vi "CallVirtualConstructorMethod.vi"(8 "error in":errorcluster, 11 "TestSuite in":refnum<class "TestSuite.lvclass">) -> (0 "error out":errorcluster, 2 "Constructor Error":errorcluster, 3 "TestSuite out":refnum<class "TestSuite.lvclass">)   [LabVIEW 2011, in "TestSuite.lvclass"]
uses:
  TestSuite.lvclass
  JKI Reuse/Filter Error Codes (Scalar)__jki_lib_error_handling -- VI Tester.vi
  Libraries/VITesterUtilities.lvlib
panel:
  # "JKI VI Tester for LabVIEW\nhttp://jkisoft.com/vi-tester\nCopyright (C) 2007-2009, JKI <info@jkisoft.com>\nALL RIGHTS RESERVED"
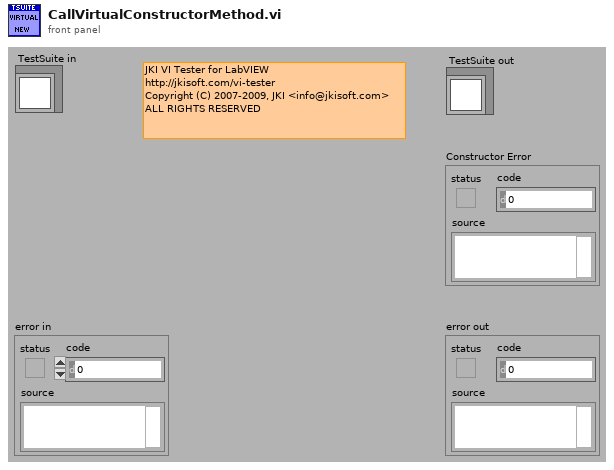
[diagram p1: front panel]
types:
  T1 = cluster{"name":string, "type desc":i16[], "flat data":string}
  T2 = cluster{"name":string, "type desc":i16[], "flat data":string}[]
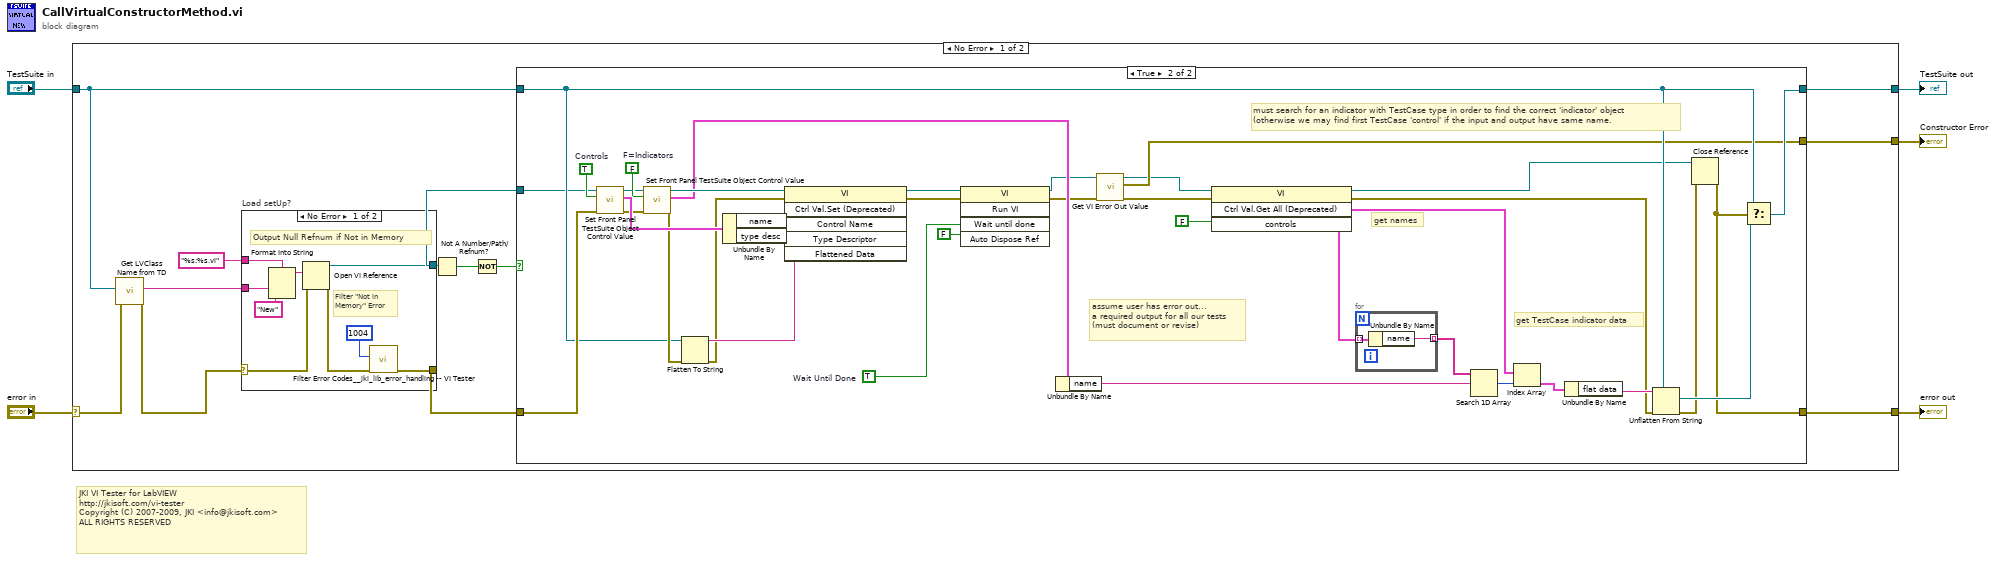
[diagram p0: block diagram]
diagram:
  # "JKI VI Tester for LabVIEW\nhttp://jkisoft.com/vi-tester\nCopyright (C) 2007-2009, JKI <info@jkisoft.com>\nALL RIGHTS RESERVED"
  n1 = case shown="No Error" "error in" {
    selector: "error in" -> [w11 w70]
    tunnel: [w17 w69] -> w1
    tunnel: [w16 _] -> w2
    tunnel: [w15 w70] -> w3
    tunnel: "TestSuite in" -> [w12 w69]
    frame No Error {
      n2 = call "Get LVClass Name from TD.vi"("error in"=w11, "Variant"=w12) -> ("error out"=w10:errorcluster, "LVClass Name"=w13:string)  [unwired: 8 in]
      n3 = case "Load setUp?" shown="No Error" w10 {
        selector: w10 -> [w21 w27]
        tunnel: [w24 _] -> w6
        tunnel: "%s:%s.vi" ("format string") -> [w23 _]
        tunnel: [w19 w27] -> w9
        tunnel: w13 -> [w22 _]
        frame No Error {
          # "Output Null Refnum if Not in Memory"
          # "Filter \"Not in Memory\" Error"
          n4 = Format Into String(format string=w23, w22, "New" ("input 2")) -> (resulting string=w25:string)  [unwired: 2 in, 1 out]
          n5 = Open VI Reference(vi path=w25, error in (no error)=w21) -> (vi reference=w24:refnum<vi>, error out=w20:errorcluster)  [unwired: 4 in]
          n6 = call-poly "Filter Error Codes__jki_lib_error_handling -- VI Tester.vi"("error in"=w20, "error code to filter"=1004) -> ("error out"=w19:errorcluster)  [unwired: 7 in, 2 out]
        }
        frame Error {
        }
      }
      n7 = Not A Number/Path/Refnum?(number/path/refnum=w6) -> (NaN/Path/Refnum?=w8:bool)
      n8 = Not(x=w8) -> (.not. x?=w7:bool)
      n9 = case shown="True" w7 {
        tunnel: [w29 w66] -> w17
        tunnel: [_ w32] -> w16
        tunnel: [w28 w36] -> w15
        tunnel: w12 -> [w29 w46]
        tunnel: w9 -> [w28 w54]
        tunnel: w6 -> [_ w35]
        frame False {
        }
        frame True {
          w51 = TRUE  # Wait Until Done
          w58 = FALSE  # F=Indicators
          w62 = TRUE  # Controls
          # "get TestCase indicator data"
          # "get names"
          # "must search for an indicator with TestCase type in order to find the correct 'indicator' object\n(otherwise we may find first TestCase 'control' if the input and output have same name."
          # "assume user has error out...\na required output for all our tests\n(must document or revise)"
          n10 = call "Set Front Panel TestSuite Object Control Value.vi"("error in"=w54, "Control (F: Indicator)"=w62, "vi reference"=w35) -> ("error out"=w57:errorcluster, "Control Value"=w61:T1, "dup vi reference"=w56:refnum<vi>)  [unwired: 5 in, 1 out]
          n11 = call "Set Front Panel TestSuite Object Control Value.vi"("error in"=w57, "Control (F: Indicator)"=w58, "vi reference"=w56) -> ("error out"=w53:errorcluster, "Control Value"=w43:T1, "dup vi reference"=w55:refnum<vi>)  [unwired: 5 in, 1 out]
          n12 = Flatten To String(anything=w46, error in (no error)=w53) -> (data string=w63:string, error out=w52:errorcluster)  [unwired: 2 in, 1 out]
          n13 = Unbundle By Name(w61) -> ("name"=w60:string, "type desc"=w59:i16[])
          n14 = invoke class="VI" method="Ctrl Val.Set (Deprecated)"(reference=w55, error in=w52, "Control Name"=w60, "Type Descriptor"=w59, "Flattened Data"=w63) -> (reference out=w65:refnum<vi>, error out=w64:errorcluster)  [unwired: 1 in, 4 out]
          n15 = invoke class="VI" method="Run VI"(reference=w65, error in=w64, "Wait until done"=w51, "Auto Dispose Ref"=FALSE ("Auto Dispose Reference")) -> (reference out=w33:refnum<vi>, error out=w34:errorcluster)  [unwired: 1 in, 3 out]
          n16 = Unbundle By Name(w43) -> ("name"=w40:string)
          n17 = call "Get VI Error Out Value.vi"("error in"=w34, "vi reference in"=w33) -> ("error out"=w30:errorcluster, "vi error out"=w32:errorcluster, "dup vi reference"=w31:refnum<vi>)  [unwired: 7 in]
          n18 = invoke class="VI" method="Ctrl Val.Get All (Deprecated)"(reference=w31, error in=w30, "controls"=FALSE ("Controls")) -> (reference out=w38:refnum<vi>, error out=w44:errorcluster, "Get All Control Values"=w42:T2)  [unwired: 1 in, 1 out]
          n19 = for {
            tunnel: w42 -> [w68] mode=indexing
            tunnel: [w67] -> w41 mode=indexing
            n20 = Unbundle By Name(w68) -> ("name"=w67:string)
          }
          n21 = Search 1D Array(1D array=w41, element=w40) -> (index of element=w49:i32)  [unwired: 1 in]
          n22 = Index Array(array=w42, index=w49) -> (element=w48:T1)
          n23 = Unbundle By Name(w48) -> ("flat data"=w47:string)
          n24 = Unflatten From String(type=w46, binary string=w47, error in (no error)=w44) -> (value=w45:refnum<class "TestSuite.lvclass">, error out=w37:errorcluster)  [unwired: 2 in, 1 out]
          n25 = Close Reference(reference=w38, error in (no error)=w37) -> (error out=w36:errorcluster)
          n26 = Select(t=w46, s=w36, f=w45) -> (s? t:f=w66:refnum<class "TestSuite.lvclass">)
        }
      }
    }
    frame Error {
    }
  }
  "error out" <- w3
  "Constructor Error" <- w2
  "TestSuite out" <- w1
